vi "write_data.vi"(8 "error in (no error)":errorcluster, 10 "data":T1, 11 "SpectralBiclustering in":refnum<class "SpectralBiclustering.lvclass">) -> (0 "error out":errorcluster, 3 "SpectralBiclustering out":refnum<class "SpectralBiclustering.lvclass">)   [LabVIEW 2020, in "SpectralBiclustering.lvclass"]
uses:
  SpectralBiclustering.lvclass
  Controls/spectral_biclustering_data.ctl
  SpectralBiclustering.lvclass/SpectralBiclustering.ctl
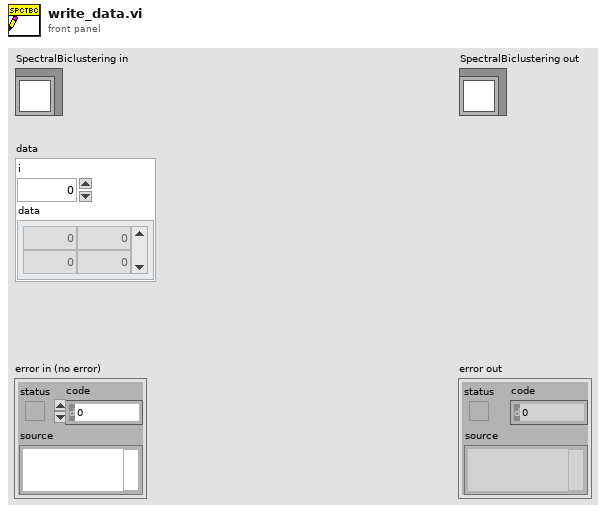
[diagram p1: front panel]
types:
  T1 = typedef "spectral_biclustering_data.ctl" = cluster{"i":dbl, "data":dbl[][]}
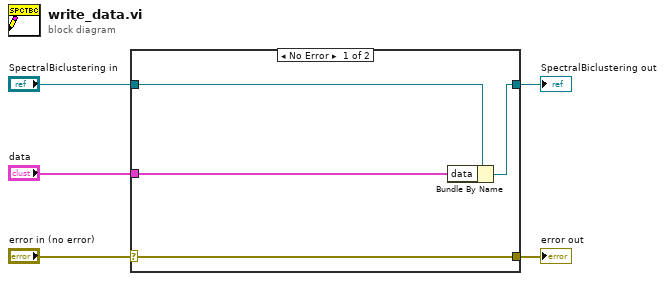
[diagram p0: block diagram]
diagram:
  n1 = case shown="No Error" "error in (no error)" {
    selector: "error in (no error)" -> [w9 w10]
    tunnel: [w9 w10] -> w4
    tunnel: [w7 w11] -> w2
    tunnel: "SpectralBiclustering in" -> [w8 w11]
    tunnel: "data" -> [w6 _]
    frame No Error {
      n2 = Bundle By Name(cluster=w8, "data"=w6) -> (w7:refnum<class "SpectralBiclustering.lvclass">)
    }
    frame Error {
    }
  }
  "error out" <- w4
  "SpectralBiclustering out" <- w2
